vi "DAQmx Counters Demo.vi"() -> ()   [LabVIEW 2025]
uses:
  <vilib>/Utility/error.llb/DialogType.ctl
  <vilib>/DAQmx/read.llb/DAQmx Read (Counter 1D DBL 1Chan NSamp).vi
  <vilib>/DAQmx/write.llb/DAQmx Write (Counter Frequency 1Chan 1Samp).vi
  <vilib>/DAQmx/create/channels.llb/DAQmx Create Channel (CO-Pulse Generation-Frequency).vi
  <vilib>/DAQmx/configure/timing.llb/DAQmx Timing (Implicit).vi
  <vilib>/DAQmx/miscellaneous.llb/DAQmx Fill In Error Info.vi
  <vilib>/DAQmx/create/channels.llb/DAQmx Create Channel (CI-Pulse Width).vi
  <vilib>/DAQmx/create/channels.llb/DAQmx Create Channel (CI-Frequency).vi
  <vilib>/DAQmx/create/channels.llb/DAQmx Create Channel (CI-Period).vi
  <resource>/objmgr/daqmx.rc
panel:
  out "Conflict Error Out":errorcluster
  out "Period":dbl[](array[numeric])
  out "Frequency":dbl[](array[numeric])
  in  "Samples per Loop":i32=1
  in  "Stop Acq":bool
  out "Pulse Width":dbl[](array[numeric])
  in  "Duty Cycle":dbl=0.5 format="%.6f"
  in  "Frequency":dbl=1.0 format="%.6f"
  in  "Stop Gen":bool
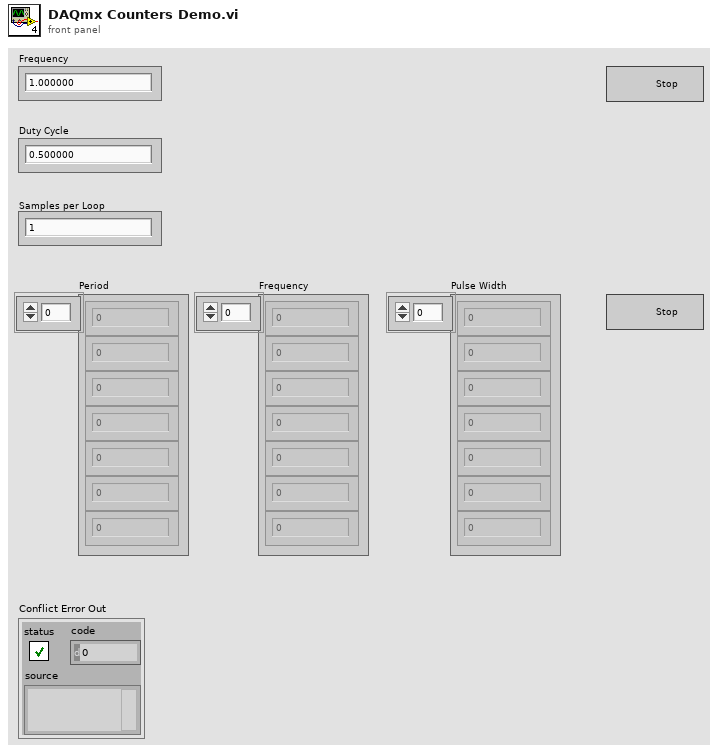
[diagram p1: front panel]
types:
  T1 = typedef "DialogType.ctl" = u16
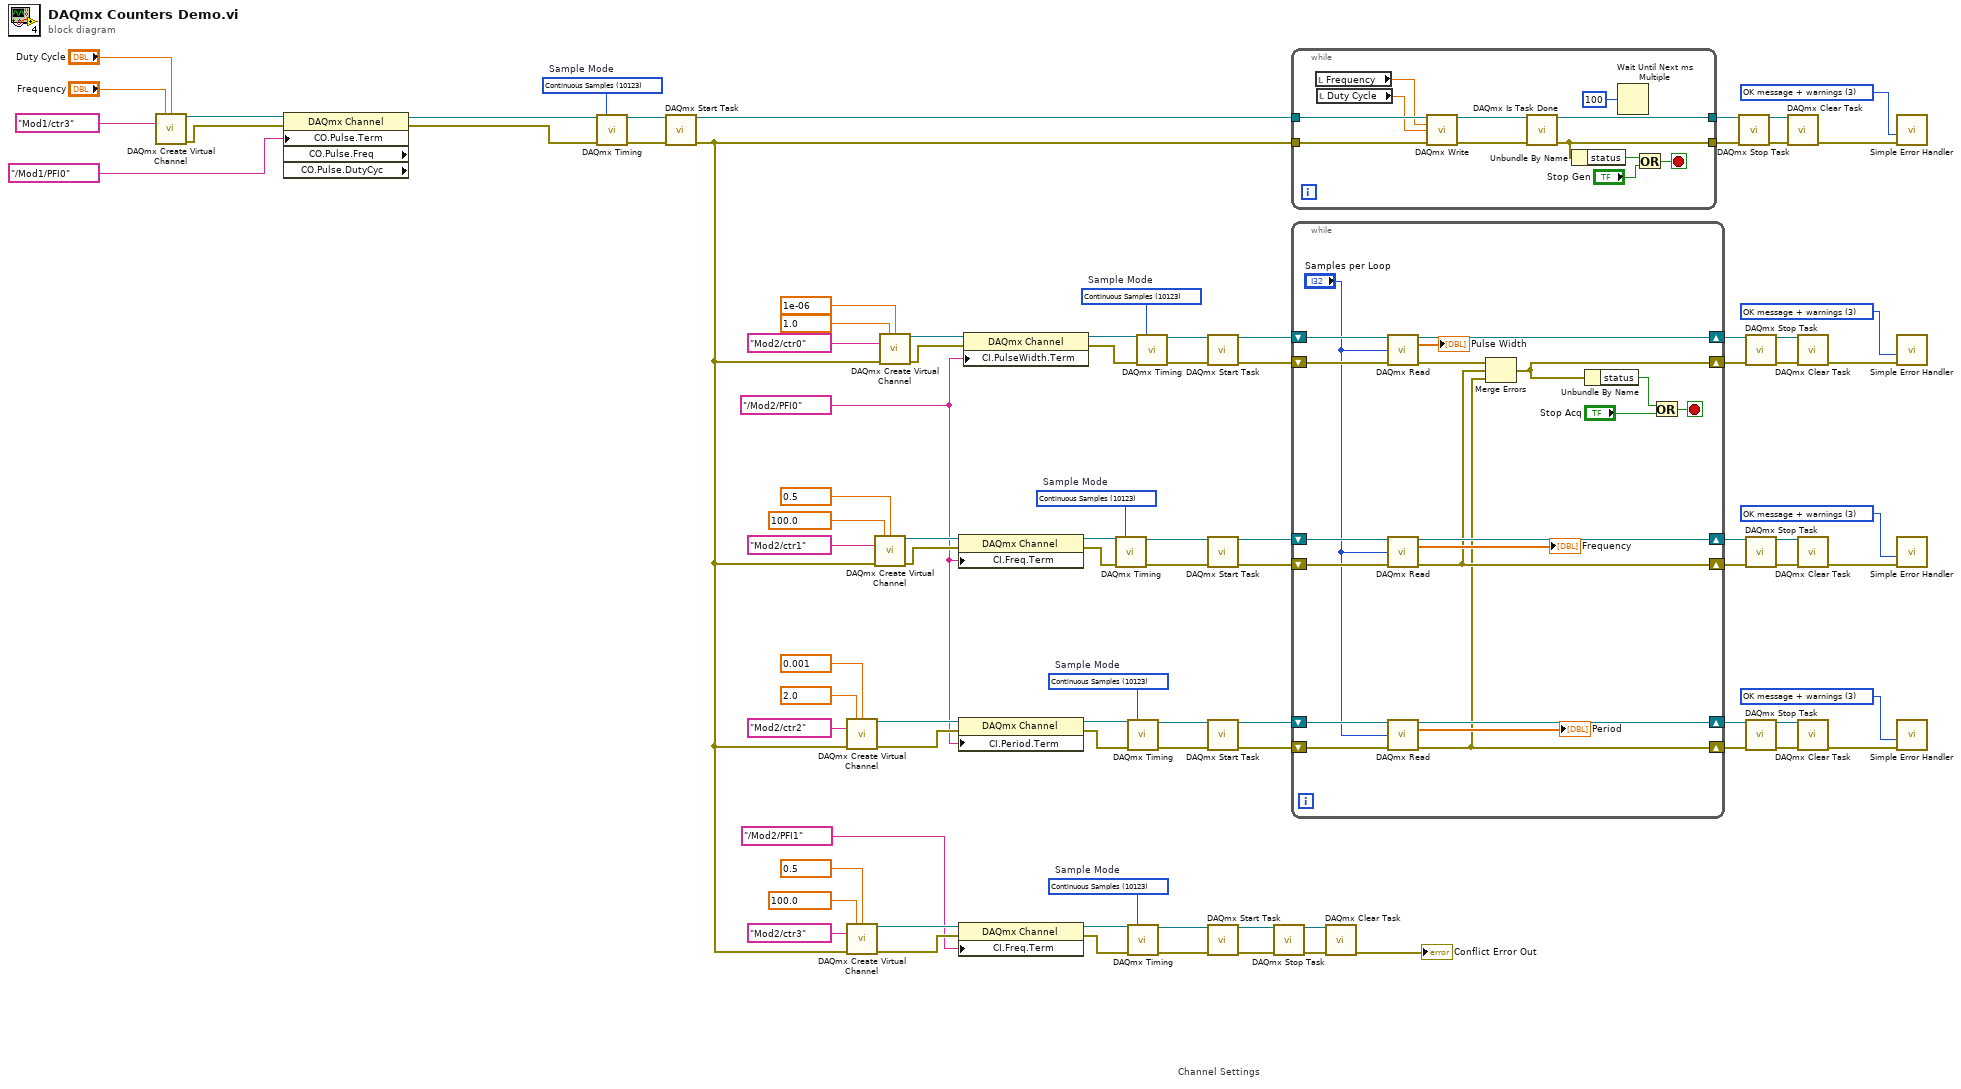
[diagram p0: block diagram]
diagram:
  w18 = 10123 items=["Finite Samples"=10178, "Continuous Samples"=10123, "Hardware Timed Single Point"=12522]  # Sample Mode
  w29 = T1 3 items=["no dialog", "OK message", "continue or stop message", "OK message + warnings", "continue/stop + warnings"] ("type of dialog (OK msg:1)")
  w40 = 10123 items=["Finite Samples"=10178, "Continuous Samples"=10123, "Hardware Timed Single Point"=12522]  # Sample Mode
  w45 = T1 3 items=["no dialog", "OK message", "continue or stop message", "OK message + warnings", "continue/stop + warnings"] ("type of dialog (OK msg:1)")
  w56 = 10123 items=["Finite Samples"=10178, "Continuous Samples"=10123, "Hardware Timed Single Point"=12522]  # Sample Mode
  w5 = tag "/Mod2/PFI0" ("Pulse Width Input Terminal")
  w61 = T1 3 items=["no dialog", "OK message", "continue or stop message", "OK message + warnings", "continue/stop + warnings"] ("type of dialog (OK msg:1)")
  w72 = 10123 items=["Finite Samples"=10178, "Continuous Samples"=10123, "Hardware Timed Single Point"=12522]  # Sample Mode
  w73 = T1 3 items=["no dialog", "OK message", "continue or stop message", "OK message + warnings", "continue/stop + warnings"] ("type of dialog (OK msg:1)")
  w90 = 10123 items=["Finite Samples"=10178, "Continuous Samples"=10123, "Hardware Timed Single Point"=12522]  # Sample Mode
  # "Channel Settings"
  n1 = call-poly <vilib>:"DAQmx Create Virtual Channel.vi"("frequency"="Frequency", "duty cycle"="Duty Cycle", "counter"=tag "Mod1/ctr3" ("Counter")) -> ("task out"=w84:refnum<k21>, "error out"=w83:errorcluster)  [unwired: 11 in]
  n2 = property class="DAQmx Channel" props=["CO.Pulse.Term", "CO.Pulse.Freq", "CO.Pulse.DutyCyc"](reference=w84, error in=w83, "CO.Pulse.Term"=tag "/Mod1/PFI0" ("Output Terminal")) -> (reference out=w80:refnum<k21>, error out=w81:errorcluster)  [unwired: 2 out]
  n3 = call-poly <vilib>:"DAQmx Timing.vi"("task/channels in"=w80, "sample mode"=w90, "error in"=w81) -> ("task out"=w85:refnum<k21>, "error out"=w86:errorcluster)  [unwired: 11 in]
  n4 = call <vilib>:"DAQmx Start Task.vi"("task/channels in"=w85, "error in"=w86) -> ("task out"=w89:refnum<k21>, "error out"=w6:errorcluster)  [unwired: 12 in]
  n5 = call-poly <vilib>:"DAQmx Create Virtual Channel.vi"("maximum value"=2.0 ("Max Frequency"), "minimum value"=0.001 ("Min Frequency"), "counter"=tag "Mod2/ctr2" ("Counter"), "error in"=w6) -> ("task out"=w28:refnum<k21>, "error out"=w27:errorcluster)  [unwired: 10 in]
  n6 = call-poly <vilib>:"DAQmx Create Virtual Channel.vi"("maximum value"=100.0 ("Max Frequency"), "minimum value"=0.5 ("Min Frequency"), "counter"=tag "Mod2/ctr3" ("Counter"), "error in"=w6) -> ("task out"=w12:refnum<k21>, "error out"=w11:errorcluster)  [unwired: 10 in]
  n7 = call-poly <vilib>:"DAQmx Create Virtual Channel.vi"("maximum value"=100.0 ("Max Frequency"), "minimum value"=0.5 ("Min Frequency"), "counter"=tag "Mod2/ctr1" ("Counter"), "error in"=w6) -> ("task out"=w44:refnum<k21>, "error out"=w43:errorcluster)  [unwired: 10 in]
  n8 = call-poly <vilib>:"DAQmx Create Virtual Channel.vi"("maximum value"=1.0 ("Max Pulse Width"), "minimum value"=1e-06 ("Min Pulse Width"), "counter"=tag "Mod2/ctr0" ("Counter"), "error in"=w6) -> ("task out"=w60:refnum<k21>, "error out"=w59:errorcluster)  [unwired: 10 in]
  n9 = property class="DAQmx Channel"(reference=w44, error in=w43, "CI.Freq.Term"=w5) -> (reference out=w54:refnum<k21>, error out=w55:errorcluster)
  n10 = property class="DAQmx Channel"(reference=w28, error in=w27, "CI.Period.Term"=w5) -> (reference out=w38:refnum<k21>, error out=w39:errorcluster)
  n11 = property class="DAQmx Channel"(reference=w12, error in=w11, "CI.Freq.Term"=tag "/Mod2/PFI1") -> (reference out=w16:refnum<k21>, error out=w17:errorcluster)
  n12 = property class="DAQmx Channel"(reference=w60, error in=w59, "CI.PulseWidth.Term"=w5) -> (reference out=w70:refnum<k21>, error out=w71:errorcluster)
  n13 = call-poly <vilib>:"DAQmx Timing.vi"("task/channels in"=w54, "sample mode"=w56, "error in"=w55) -> ("task out"=w22:refnum<k21>, "error out"=w21:errorcluster)  [unwired: 11 in]
  n14 = call-poly <vilib>:"DAQmx Timing.vi"("task/channels in"=w38, "sample mode"=w40, "error in"=w39) -> ("task out"=w20:refnum<k21>, "error out"=w19:errorcluster)  [unwired: 11 in]
  n15 = call-poly <vilib>:"DAQmx Timing.vi"("task/channels in"=w16, "sample mode"=w18, "error in"=w17) -> ("task out"=w8:refnum<k21>, "error out"=w7:errorcluster)  [unwired: 11 in]
  n16 = call-poly <vilib>:"DAQmx Timing.vi"("task/channels in"=w70, "sample mode"=w72, "error in"=w71) -> ("task out"=w24:refnum<k21>, "error out"=w23:errorcluster)  [unwired: 11 in]
  n17 = call <vilib>:"DAQmx Start Task.vi"("task/channels in"=w24, "error in"=w23) -> ("task out"=w69:refnum<k21>, "error out"=w68:errorcluster)  [unwired: 12 in]
  n18 = call <vilib>:"DAQmx Start Task.vi"("task/channels in"=w22, "error in"=w21) -> ("task out"=w53:refnum<k21>, "error out"=w52:errorcluster)  [unwired: 12 in]
  n19 = call <vilib>:"DAQmx Start Task.vi"("task/channels in"=w20, "error in"=w19) -> ("task out"=w37:refnum<k21>, "error out"=w36:errorcluster)  [unwired: 12 in]
  n20 = call <vilib>:"DAQmx Start Task.vi"("task/channels in"=w8, "error in"=w7) -> ("task out"=w1:refnum<k21>, "error out"=w2:errorcluster)  [unwired: 12 in]
  n21 = call <vilib>:"DAQmx Stop Task.vi"("task/channels in"=w1, "error in"=w2) -> ("task out"=w14:refnum<k21>, "error out"=w13:errorcluster)  [unwired: 12 in]
  n22 = while {
    tunnel: w89 -> [w96]
    tunnel: w6 -> [w95]
    tunnel: [w100] -> w74
    tunnel: [w101] -> w75
    stop <- w102 stop-if-true
    n23 = local read "Frequency"() -> (w91:dbl)
    n24 = local read "Duty Cycle"() -> (w92:dbl)
    n25 = call-poly <vilib>:"DAQmx Write.vi"("task/channels in"=w96, "frequency"=w91, "duty cycle"=w92, "error in"=w95) -> ("task out"=w94:refnum<k21>, "error out"=w93:errorcluster)  [unwired: 9 in, 1 out]
    n26 = call <vilib>:"DAQmx Is Task Done.vi"("task/channels in"=w94, "error in"=w93) -> ("task out"=w101:refnum<k21>, "error out"=w100:errorcluster)  [unwired: 11 in, 1 out]
    n27 = Unbundle By Name(w100) -> ("status"=w99:bool)
    n28 = Wait Until Next ms Multiple(millisecond multiple=u32 100) -> ()  [unwired: 1 out]
    n29 = Or(x=w99, y="Stop Gen") -> (x .or. y?=w102:bool)
  }
  n30 = while {
    shift-right: [w120] -> w63
    shift-left: w69 -> [w122]
    shift-right: [w108] -> w62
    shift-left: w68 -> [w121]
    shift-right: [w116] -> w47
    shift-left: w53 -> [w118]
    shift-right: [w104] -> w46
    shift-left: w52 -> [w117]
    shift-right: [w113] -> w31
    shift-left: w37 -> [w115]
    shift-right: [w103] -> w30
    shift-left: w36 -> [w114]
    stop <- w107 stop-if-true
    n31 = call-poly <vilib>:"DAQmx Read.vi"("task/channels in"=w122, "number of samples per channel"="Samples per Loop", "error in"=w121) -> ("task out"=w120:refnum<k21>, "data"=→"Pulse Width":dbl[], "error out"=w119:errorcluster)  [unwired: 10 in]
    n32 = call-poly <vilib>:"DAQmx Read.vi"("task/channels in"=w118, "number of samples per channel"="Samples per Loop", "error in"=w117) -> ("task out"=w116:refnum<k21>, "data"=→"Frequency":dbl[], "error out"=w104:errorcluster)  [unwired: 10 in]
    n33 = call-poly <vilib>:"DAQmx Read.vi"("task/channels in"=w115, "number of samples per channel"="Samples per Loop", "error in"=w114) -> ("task out"=w113:refnum<k21>, "data"=→"Period":dbl[], "error out"=w103:errorcluster)  [unwired: 10 in]
    n34 = Merge Errors(w119, w104, w103) -> (w108:errorcluster)
    n35 = Unbundle By Name(w108) -> ("status"=w111:bool)
    n36 = Or(x=w111, y="Stop Acq") -> (x .or. y?=w107:bool)
  }
  n37 = call <vilib>:"DAQmx Clear Task.vi"("task in"=w14, "error in"=w13) -> ("error out"=→"Conflict Error Out":errorcluster)  [unwired: 13 in]
  n38 = call <vilib>:"DAQmx Stop Task.vi"("task/channels in"=w75, "error in"=w74) -> ("task out"=w77:refnum<k21>, "error out"=w76:errorcluster)  [unwired: 12 in]
  n39 = call <vilib>:"DAQmx Stop Task.vi"("task/channels in"=w63, "error in"=w62) -> ("task out"=w65:refnum<k21>, "error out"=w64:errorcluster)  [unwired: 12 in]
  n40 = call <vilib>:"DAQmx Stop Task.vi"("task/channels in"=w47, "error in"=w46) -> ("task out"=w49:refnum<k21>, "error out"=w48:errorcluster)  [unwired: 12 in]
  n41 = call <vilib>:"DAQmx Stop Task.vi"("task/channels in"=w31, "error in"=w30) -> ("task out"=w33:refnum<k21>, "error out"=w32:errorcluster)  [unwired: 12 in]
  n42 = call <vilib>:"DAQmx Clear Task.vi"("task in"=w77, "error in"=w76) -> ("error out"=w88:errorcluster)  [unwired: 13 in]
  n43 = call <vilib>:"DAQmx Clear Task.vi"("task in"=w65, "error in"=w64) -> ("error out"=w67:errorcluster)  [unwired: 13 in]
  n44 = call <vilib>:"DAQmx Clear Task.vi"("task in"=w49, "error in"=w48) -> ("error out"=w51:errorcluster)  [unwired: 13 in]
  n45 = call <vilib>:"DAQmx Clear Task.vi"("task in"=w33, "error in"=w32) -> ("error out"=w35:errorcluster)  [unwired: 13 in]
  n46 = call <vilib>:"Simple Error Handler.vi"("type of dialog (OK msg:1)"=w73, "error in (no error)"=w88) -> ()  [unwired: 3 in, 5 out]
  n47 = call <vilib>:"Simple Error Handler.vi"("type of dialog (OK msg:1)"=w61, "error in (no error)"=w67) -> ()  [unwired: 3 in, 5 out]
  n48 = call <vilib>:"Simple Error Handler.vi"("type of dialog (OK msg:1)"=w45, "error in (no error)"=w51) -> ()  [unwired: 3 in, 5 out]
  n49 = call <vilib>:"Simple Error Handler.vi"("type of dialog (OK msg:1)"=w29, "error in (no error)"=w35) -> ()  [unwired: 3 in, 5 out]
